vi "XNET Stop.vi"(0 "session in":refnum<k21>, 5 "scope (normal)":T1 items=["Normal", "Session Only", "Interface Only", "Session Only Blocking"], 11 "error in (no error)":errorcluster) -> (4 "session out":refnum<k21>, 15 "error out":errorcluster)   [LabVIEW 2018]
doc: "Stops communication for the specified XNET session."
uses:
  XNET Control Scope.ctl
  nixlvapi.dll
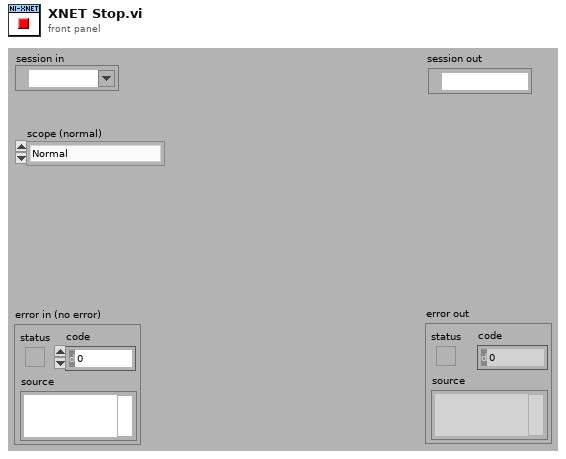
[diagram p1: front panel]
types:
  T1 = typedef "XNET Control Scope.ctl" = u32
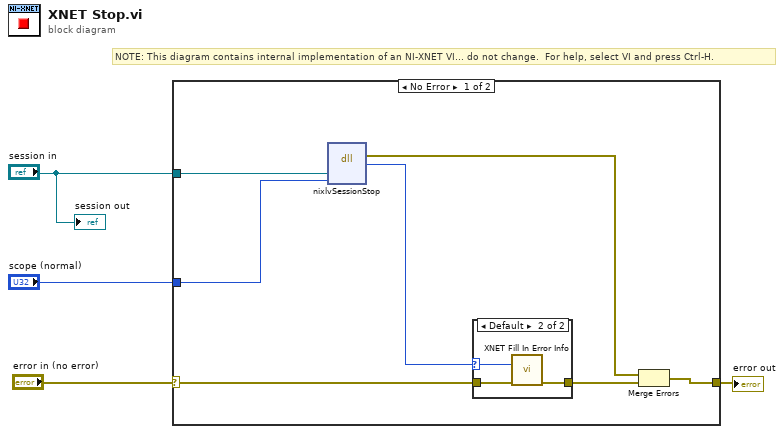
[diagram p0: block diagram]
diagram:
  # "NOTE: This diagram contains internal implementation of an NI-XNET VI... do not change.  For help, select VI and press Ctrl-H."
  n1 = case shown="No Error" "error in (no error)" {
    selector: "error in (no error)" -> [w10 w16]
    tunnel: "session in" -> [w11 _]
    tunnel: [w6 w16] -> w4
    tunnel: "scope (normal)" -> [w7 _]
    frame No Error {
      # "NOTE: This diagram contains internal implementation of an NI-XNET VI... do not change.  For help, select VI and press Ctrl-H."
      n2 = dll-call lib="nixlvapi.*" fn="nixlvSessionStop" ("nilvxaiu.dll:lvxenSessionClear")("reference"=w11, "scope"=w7) -> (error out=w5:errorcluster, "return type"=w8:i32)  [unwired: 4 in, 2 out]
      n3 = case shown="Default" w8 {
        selector: w8 -> [_ w13]
        tunnel: w10 -> [w12 w14]
        tunnel: [w12 w15] -> w9
        frame 0 {
        }
        frame Default {
          n4 = call "XNET Fill In Error Info.vi"("status code"=w13, "error in"=w14) -> ("error out"=w15:errorcluster)  [unwired: 13 out]
        }
      }
      n5 = Merge Errors(w5, w9) -> (w6:errorcluster)
    }
    frame Error {
    }
  }
  "error out" <- w4
  "session out" <- "session in"
